vi "Data Logging in Autonomous.vi"() -> ()   [LabVIEW 2011]
uses:
  <vilib>/Utility/file.llb/Write To Spreadsheet File (DBL).vi
panel:
  out "array 4":dbl[][](array[numeric])
  out "array 3":dbl[][](array[numeric])
  out "array 2":dbl[][](array[numeric])
  in  "Save Data 2":bool
  out "array":dbl[][](array[numeric])
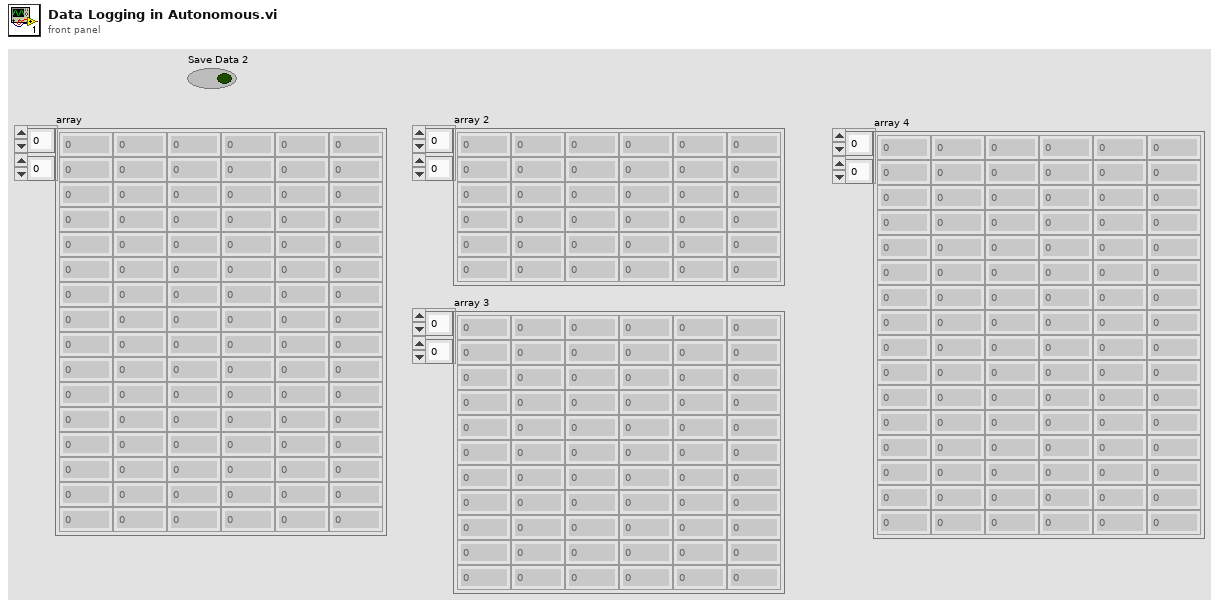
[diagram p1: front panel]
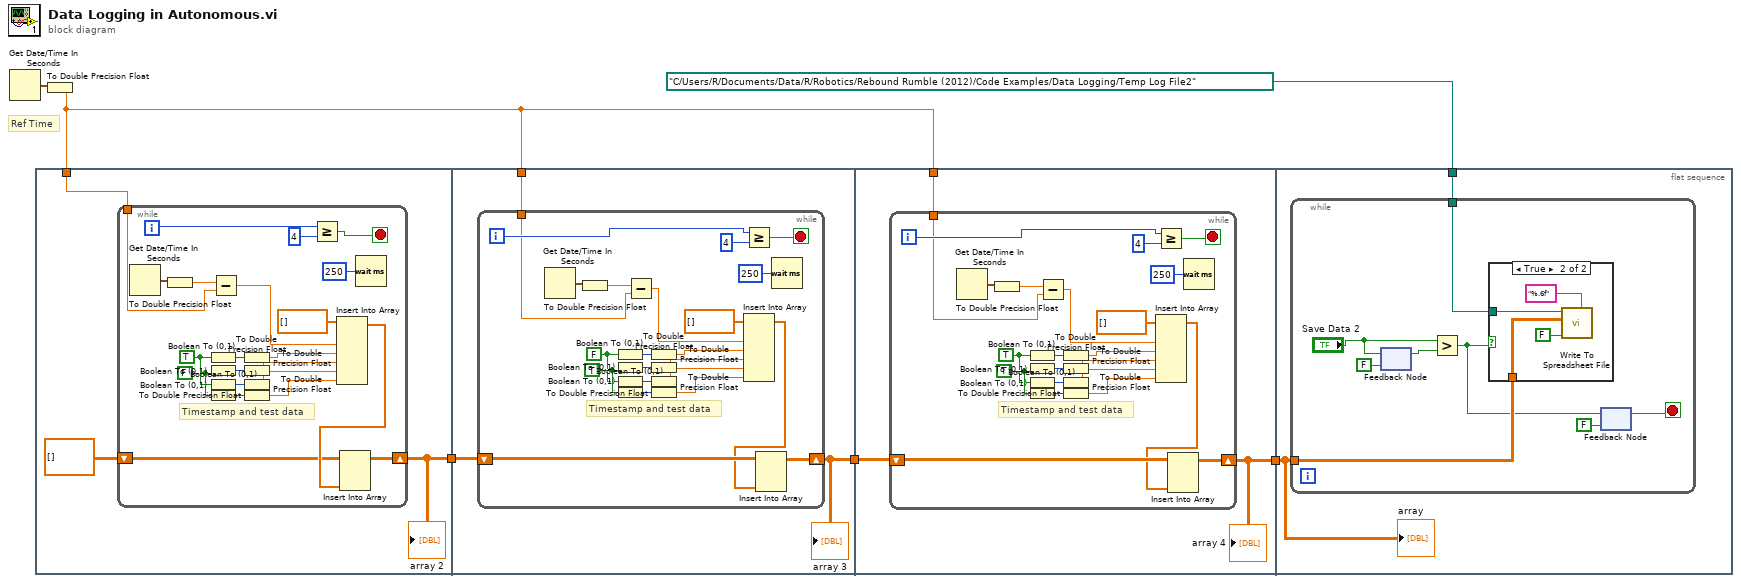
[diagram p0: block diagram]
diagram:
  # "Ref Time"
  n1 = Get Date/Time In Seconds() -> (seconds since 1Jan1904=w6:timestamp)
  n2 = flat-sequence {
    tunnel: w4 -> [w9]
    tunnel: [w7] -> w5
    tunnel: w5 -> [w34]
    tunnel: w4 -> [w33]
    tunnel: [w32] -> w3
    tunnel: w4 -> [w59]
    tunnel: w3 -> [w58]
    tunnel: [w57] -> w2
    tunnel: w2 -> [w82]
    tunnel: path "C:/Users/R/Documents/Data/R/Robotics/Rebound Rumble (2012)/Code Examples/Data Logging/Temp Log File2" ("datalog path (use dialog)") -> [w83]
    frame #0 {
      n3 = while {
        tunnel: w9 -> [w13]
        shift-right: [w10] -> w7
        shift-left: dbl[][] [] ("array") -> [w11]
        i -> [w30]
        stop <- w31 stop-if-true
        w15 = FALSE
        w16 = TRUE ("Boolean")
        # "Timestamp and test data"
        n4 = Get Date/Time In Seconds() -> (seconds since 1Jan1904=w23:timestamp)
        n5 = To Double Precision Float(number=w23) -> (double precision float=w22:dbl)
        n6 = Boolean To (0,1)(Boolean=w16) -> (0, 1=w24:i16)
        n7 = Boolean To (0,1)(Boolean=w15) -> (0, 1=w25:i16)
        n8 = Boolean To (0,1)(Boolean=w16) -> (0, 1=w27:i16)
        n9 = Boolean To (0,1)(Boolean=w15) -> (0, 1=w26:i16)
        n10 = Subtract(x=w22, y=w13) -> (x-y=w18:dbl)
        n11 = To Double Precision Float(number=w24) -> (double precision float=w21:dbl)
        n12 = To Double Precision Float(number=w25) -> (double precision float=w20:dbl)
        n13 = To Double Precision Float(number=w27) -> (double precision float=w14:dbl)
        n14 = To Double Precision Float(number=w26) -> (double precision float=w17:dbl)
        n15 = Greater Or Equal?(x=w30, y=4) -> (x >= y?=w31:bool)
        n16 = Insert Into Array(array=dbl[] [], new element #1=w18, new element #2=w21, new element #3=w20, new element #4=w14, new element #5=w17) -> (w12:dbl[])  [unwired: 1 in]
        n17 = Insert Into Array(array=w11, new element=w12) -> (w10:dbl[][])  [unwired: 2 in]
        n18 = Wait (ms)(milliseconds to wait=u32 250) -> ()  [unwired: 1 out]
      }
      "array 2" <- w7
    }
    frame #1 {
      n19 = while {
        tunnel: w33 -> [w38]
        shift-right: [w36] -> w32
        shift-left: w34 -> [w37]
        i -> [w54]
        stop <- w55 stop-if-true
        w51 = TRUE
        w50 = FALSE ("Boolean")
        # "Timestamp and test data"
        n20 = Get Date/Time In Seconds() -> (seconds since 1Jan1904=w40:timestamp)
        n21 = To Double Precision Float(number=w40) -> (double precision float=w41:dbl)
        n22 = Boolean To (0,1)(Boolean=w50) -> (0, 1=w46:i16)
        n23 = Boolean To (0,1)(Boolean=w51) -> (0, 1=w45:i16)
        n24 = Boolean To (0,1)(Boolean=w50) -> (0, 1=w43:i16)
        n25 = Boolean To (0,1)(Boolean=w51) -> (0, 1=w44:i16)
        n26 = Subtract(x=w41, y=w38) -> (x-y=w39:dbl)
        n27 = To Double Precision Float(number=w46) -> (double precision float=w47:dbl)
        n28 = To Double Precision Float(number=w45) -> (double precision float=w48:dbl)
        n29 = To Double Precision Float(number=w43) -> (double precision float=w52:dbl)
        n30 = To Double Precision Float(number=w44) -> (double precision float=w49:dbl)
        n31 = Greater Or Equal?(x=w54, y=4) -> (x >= y?=w55:bool)
        n32 = Insert Into Array(array=dbl[] [], new element #1=w39, new element #2=w47, new element #3=w48, new element #4=w52, new element #5=w49) -> (w35:dbl[])  [unwired: 1 in]
        n33 = Insert Into Array(array=w37, new element=w35) -> (w36:dbl[][])  [unwired: 2 in]
        n34 = Wait (ms)(milliseconds to wait=u32 250) -> ()  [unwired: 1 out]
      }
      "array 3" <- w32
    }
    frame #2 {
      n35 = while {
        tunnel: w59 -> [w63]
        shift-right: [w61] -> w57
        shift-left: w58 -> [w62]
        i -> [w79]
        stop <- w80 stop-if-true
        w76 = TRUE
        w75 = TRUE ("Boolean")
        # "Timestamp and test data"
        n36 = Get Date/Time In Seconds() -> (seconds since 1Jan1904=w65:timestamp)
        n37 = To Double Precision Float(number=w65) -> (double precision float=w66:dbl)
        n38 = Boolean To (0,1)(Boolean=w75) -> (0, 1=w71:i16)
        n39 = Boolean To (0,1)(Boolean=w76) -> (0, 1=w70:i16)
        n40 = Boolean To (0,1)(Boolean=w75) -> (0, 1=w68:i16)
        n41 = Boolean To (0,1)(Boolean=w76) -> (0, 1=w69:i16)
        n42 = Subtract(x=w66, y=w63) -> (x-y=w64:dbl)
        n43 = To Double Precision Float(number=w71) -> (double precision float=w72:dbl)
        n44 = To Double Precision Float(number=w70) -> (double precision float=w73:dbl)
        n45 = To Double Precision Float(number=w68) -> (double precision float=w77:dbl)
        n46 = To Double Precision Float(number=w69) -> (double precision float=w74:dbl)
        n47 = Greater Or Equal?(x=w79, y=4) -> (x >= y?=w80:bool)
        n48 = Insert Into Array(array=dbl[] [], new element #1=w64, new element #2=w72, new element #3=w73, new element #4=w77, new element #5=w74) -> (w60:dbl[])  [unwired: 1 in]
        n49 = Insert Into Array(array=w62, new element=w60) -> (w61:dbl[][])  [unwired: 2 in]
        n50 = Wait (ms)(milliseconds to wait=u32 250) -> ()  [unwired: 1 out]
      }
      "array 4" <- w57
    }
    frame #3 {
      n51 = while {
        tunnel: w83 -> [w88]
        tunnel: w82 -> [w87]
        stop <- w85 stop-if-true
        n52 = feedback #1(FALSE ("Save Data")) -> (w91:bool)
        n53 = feedback-in #1("Save Data 2") -> ()
        n54 = Greater?(x="Save Data 2", y=w91) -> (0:w86:bool)
        n55 = case shown="True" w86 {
          tunnel: w88 -> [_ w95]
          tunnel: w87 -> [_ w93]
          frame False {
          }
          frame True {
            n56 = call-poly <vilib>:"Write To Spreadsheet File.vi"("format (%.3f)"="%.6f", "append to file? (new file:F)"=FALSE, "2D data"=w93, "file path (dialog if empty)"=w95) -> ()  [unwired: 2 in, 3 out]
          }
        }
        n57 = feedback-in #2(w86) -> ()
        n58 = feedback #2(FALSE) -> (w85:bool)
      }
      "array" <- w82
    }
  }
  n59 = To Double Precision Float(number=w6) -> (double precision float=w4:dbl)
